vi "Set message.vi"(10 "wamplv.lvlib:WampMessage MsgPack.lvclass":refnum<class "WampMessage MsgPack.lvclass">, 11 "WelcomeHandler MsgPack in":refnum<class "WelcomeHandler MsgPack.lvclass">) -> (3 "WelcomeHandler MsgPack out":refnum<class "WelcomeHandler MsgPack.lvclass">)   [LabVIEW 2020, in "wamplv.lvlib" / "WelcomeHandler MsgPack.lvclass"]
uses:
  WelcomeHandler MsgPack.lvclass
  WelcomeHandler MsgPack.lvclass/WelcomeHandler MsgPack.ctl
  SerialisedMessages/MsgPackMessage/WampMessage MsgPack.lvclass
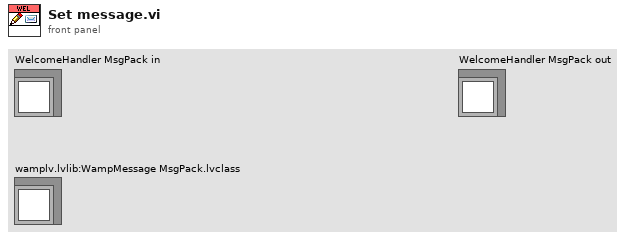
[diagram p1: front panel]
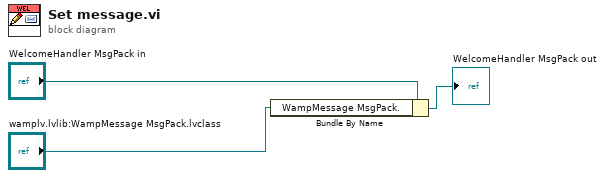
[diagram p0: block diagram]
diagram:
  n1 = Bundle By Name(cluster="WelcomeHandler MsgPack in", "WampMessage MsgPack."="wamplv.lvlib:WampMessage MsgPack.lvclass") -> (→"WelcomeHandler MsgPack out":refnum<class "WelcomeHandler MsgPack.lvclass">)
